vi "Host__MainNewS.vi"() -> ()   [LabVIEW 2018]
uses:
  Type_Def/Type_Def ControlState.ctl
  Type_Def/Type_Def Actuator Controls.ctl
  Type_Def/Master_DataControl.ctl
  Type_Def/TypeDef_cRIODatas.ctl
  Type_Def/Type_Def IMUDatas.ctl
  Type_Def/TypeDef_BMSDatas.ctl
  Type_Def/TypeDef_BMSStatuss.ctl
  Type_Def/TypeDef FixedMotorData.ctl
  <vilib>/Platform/TimedLoop/XDataNode/timing_clust.ctl
  <vilib>/Platform/TimedLoop/XDataNode/nitl_modes.ctl
  <vilib>/Platform/TimedLoop/XDataNode/wakeup.ctl
  <vilib>/Utility/file.llb/Write Delimited Spreadsheet (string).vi
  <vilib>/platform/TimedLoop/XDataNode/XDataNode.xnode
  HealthCheckClass/HealthCheck.lvclass
  <vilib>/Platform/TimedLoop/XDataNode/XDNodeRunTimeDep.lvlib
panel:
  in  "Simulate data":bool
  in  "Simulate Data\nChange values":bool
  out "Fault indicator":bool
  in  "Shutdown":bool
  out "Shorting to\n Chassis":bool
  out "High voltage\nat Contacts":bool
  out "Precharge Indicator":bool
  out "High Side":bool
  out "Vent Indicator":bool
  out "Pump Indicator":bool
  out "Reverse Indicator":bool
  out "Enum":T1
  out "Brake Indicator":bool
  out "Low Side":bool
  out "Forward Indicator":bool
  out "EMCY Brake":bool
  out "24V Power":bool
  out "x Acceleration (g)":dbl(graph)
  out "Speed (mph)":dbl(graph)
  in  "ForceIdle":bool
  in  "stop":bool
  out "HealthCheckTable":string[][](table)
  in  "Tab Control":T2(tab)
  in  "Service Push RPM target":i16=50
  in  "DrvieEnable":bool
  in  "ServiceHOLD":bool
  in  "Service Toggle":bool
  in  "Systems check\nRPM target":i16=50
  in  "Disable Fault \nCheck":bool
  in  "Vent (SC)":bool
  in  "Low Side (SC)":bool
  in  "SystemsCheck enabler":bool caption="High\nSide"
  in  "Brakes (SC)":bool
  in  "Pump (SC)":bool
  in  "Forward (SC)":bool
  in  "Reverse (SC)":bool
  in  "Pre-Charge (SC)":bool
  in  "High Side (SC)":bool
  in  "DriveEnable(SC)":bool
  in  "Release Fault":bool
  in  "Vent":bool
  in  "Ready":bool
  in  "Launch":bool
  out "Braking time (ms)":dbl
  out "Crawling time (ms)":dbl
  out "Crawling Precharge time (ms)":dbl
  out "Pushing time (ms)":dbl
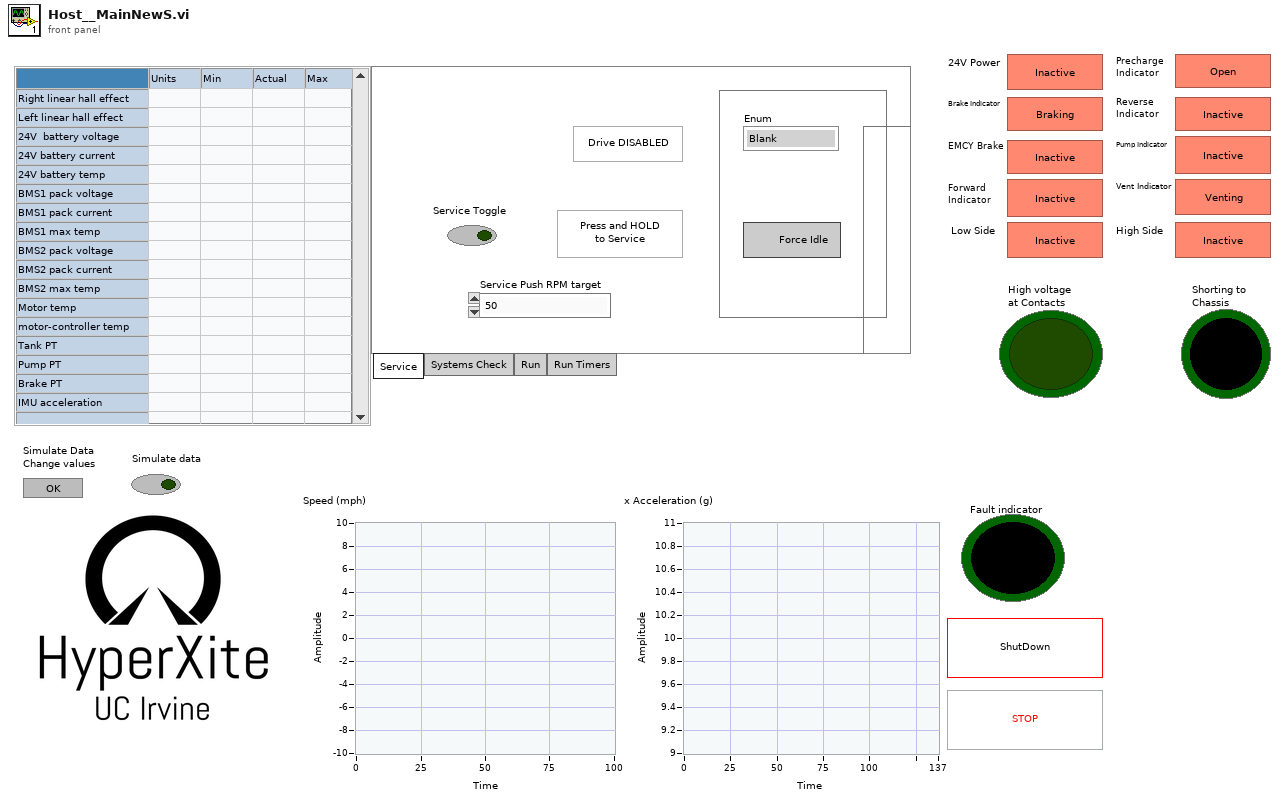
[diagram p1: front panel]
types:
  T1 = typedef "Type_Def ControlState.ctl" = enum16{"Blank", "Systems Check", "Idle", "Ready", "Pushing", "CrawlingPrecharge", "Braking", "Fault", "Boot Up", "Crawling", "Shutdown", "Service Push", "Service Wait", "Vent", "Precharge"}
  T2 = enum32{"Service", "Systems Check", "Run", "Run Timers"}
  T3 = enum8{"Enabled", "Disabled", "Disabled and Grayed Out"}
  T4 = typedef "Type_Def Actuator Controls.ctl" = cluster{"Reverse ":bool, "Precharge Ctrl":bool, "Pump Ctrl":bool, "24 VDC Ctr":bool, "Vent Solenoid":bool, "Brake Solenoid":bool, "EMCY  Brake Solenoid":bool, "Digital Out 7B ":bool, "Forward Ctrl":bool, " Contact H2":bool, "Contact L2":bool, "LED RED":bool, "LED GREEN":bool, " Digital Out 7A":bool, " Contact H1":bool, "Contact L1":bool}
  T5 = typedef "Master_DataControl.ctl" = cluster{"cRIO Data":T6, "IMU Data":T7, "BMS Data":T8, "Motor Data":T10}
  T6 = typedef "TypeDef_cRIODatas.ctl" = cluster{"HallEffect Right (cm)":dbl, "HallEffect Left (cm)":dbl, "Optical Sensor 1 (V)":dbl, "Optical Sensor 2 (V)":dbl, "24V Voltage  (V)":dbl, "24V Current (A)":dbl, "Contactor H1 Continuity":dbl, "Contactor L1 Continuity ":dbl, "Contactor H2 Continuity":dbl, "Contactor L2 Continuity ":dbl, "Brake PT(psig)":dbl, "Pump PT (psig)":dbl, "24V Temp   (C)":dbl, "Tank PT(psig) ":dbl, "ABS Pressure 1 (psig)":dbl, "ABS Pressure 2 (psig) ":dbl, "Displacement (ft)":dbl, "Velocity (ft/s)":dbl, "Time (ms)":dbl, "PV 1 Temp":dbl, "PV2 Temp":dbl}
  T7 = typedef "Type_Def IMUDatas.ctl" = cluster{"y acceleration (g)":dbl, "Pressure (psia)":dbl, "Temperature (F)":dbl}
  T8 = typedef "TypeDef_BMSDatas.ctl" = cluster{"Pack 1 Max Cell\n Voltage (V)":dbl, "Pack 1 Max Cell\n ID ":dbl, "Pack 1 Min Cell \nVoltage (V)":dbl, "Pack 1 Min Cell \nID ":dbl, "Pack 1 State of Charge  (%)":dbl, "Pack 1 Average Voltage1 (V)":dbl, "Pack 1Voltage Delta (V)":dbl, "Pack 1 Current (A)":dbl, "Pack 1 Voltage (V)":dbl, "Pack 1 Max Resistance (Ohm)":dbl, "Pack 1Min Resistance (Ohm)":dbl, "Pack 1Average Resistance (Ohm)":dbl, "Pack 1Delta Resistance (Ohm)":dbl, "Pack 1 Highest Temperature(F)":dbl, "BmsStatus1":T9, "Pack 2 Max Cell\n Voltage (V) ":dbl, "Pack 2 Max Cell\n ID  ":dbl, "Pack 2 Min Cell \nVoltage (V) ":dbl, "Pack 2 Min Cell \nID  ":dbl, "Pack 2 Average Voltage1 (V)":dbl, "Pack 2 Voltage Delta (V) ":dbl, "Pack 2 Current (A)":dbl, "Pack 2 Voltage (V) ":dbl, "Pack 2 State of Charge  (%) ":dbl, "Pack 2 Max Resistance (Ohm) ":dbl, "Pack 2 Min Resistance (Ohm)":dbl, "Pack 2 Average Resistance (Ohm)":dbl, "Pack 2 Delta Resistance (Ohm) ":dbl, "Pack 2 Highest Temperature(F) ":dbl, "BmsStatus 2":T9}
  T9 = typedef "TypeDef_BMSStatuss.ctl" = cluster{"isFault":bool, "isolationMonitoring":bool}
  T10 = typedef "TypeDef FixedMotorData.ctl" = cluster{" Velocity (RPM)":dbl, " MotorTemp(C)":dbl, " ControlTemp(C)":dbl, " DcLinkVolt(V)":dbl, " ErrorCode":dbl, "IsAlive":bool, "motorStatus":cluster{"isReady":bool, "isOn":bool, "isOperEn":bool, "isFault":bool, "isVoltEn":bool, "targetReached":bool, "isWarning":bool}, "motorControllerState":u16}
  T11 = typedef "XDNodeRunTimeDep.lvlib/timing_clust.ctl" = cluster{"Expected End [f-1]":u64, "Actual End [f-1]":u64, "Finished Late? [f-1]":bool, "Expected End [i-1]":u64, "Actual End [i-1]":u64, "Finished Late? [i-1]":bool, "Expected Start [i]":u64, "Actual Start [i]":u64, "Expected Start [f]":u64, "Actual Start [f]":u64, "Source Name":string, "Structure Name":string, "Period":i64, "Deadline":i64, "Offset":i64, "Start":i64, "Priority":i32, "Timeout":i32, "Mode":T12, "Wakeup Reason":T13, "Error":errorcluster, "Source Type":string, "Secondary Source Type":string, "Global End Time":u64, "Global Start Time":u64, "Frame Duration":u64, "Iteration Duration":u64, "Assigned CPU":i32, "I/O Scan Engine Mode":u32}
  T12 = typedef "XDNodeRunTimeDep.lvlib/nitl_modes.ctl" = enum32{"No Change", "Process missed periods, maintain original phase", "Discard missed periods, maintain original phase", "Process missed periods, ignore original phase", "Discard missed periods, ignore original phase"}
  T13 = typedef "XDNodeRunTimeDep.lvlib/wakeup.ctl" = enum32{"Normal", "Aborted", "Asynchronous wakeup", "Timing source error", "Timed loop error", "Timeout"}
  T14 = typedef "HealthCheck.lvclass/HCState_TypeDef.ctl" = enum16{"Initialization", "Running", "Modify Table"}
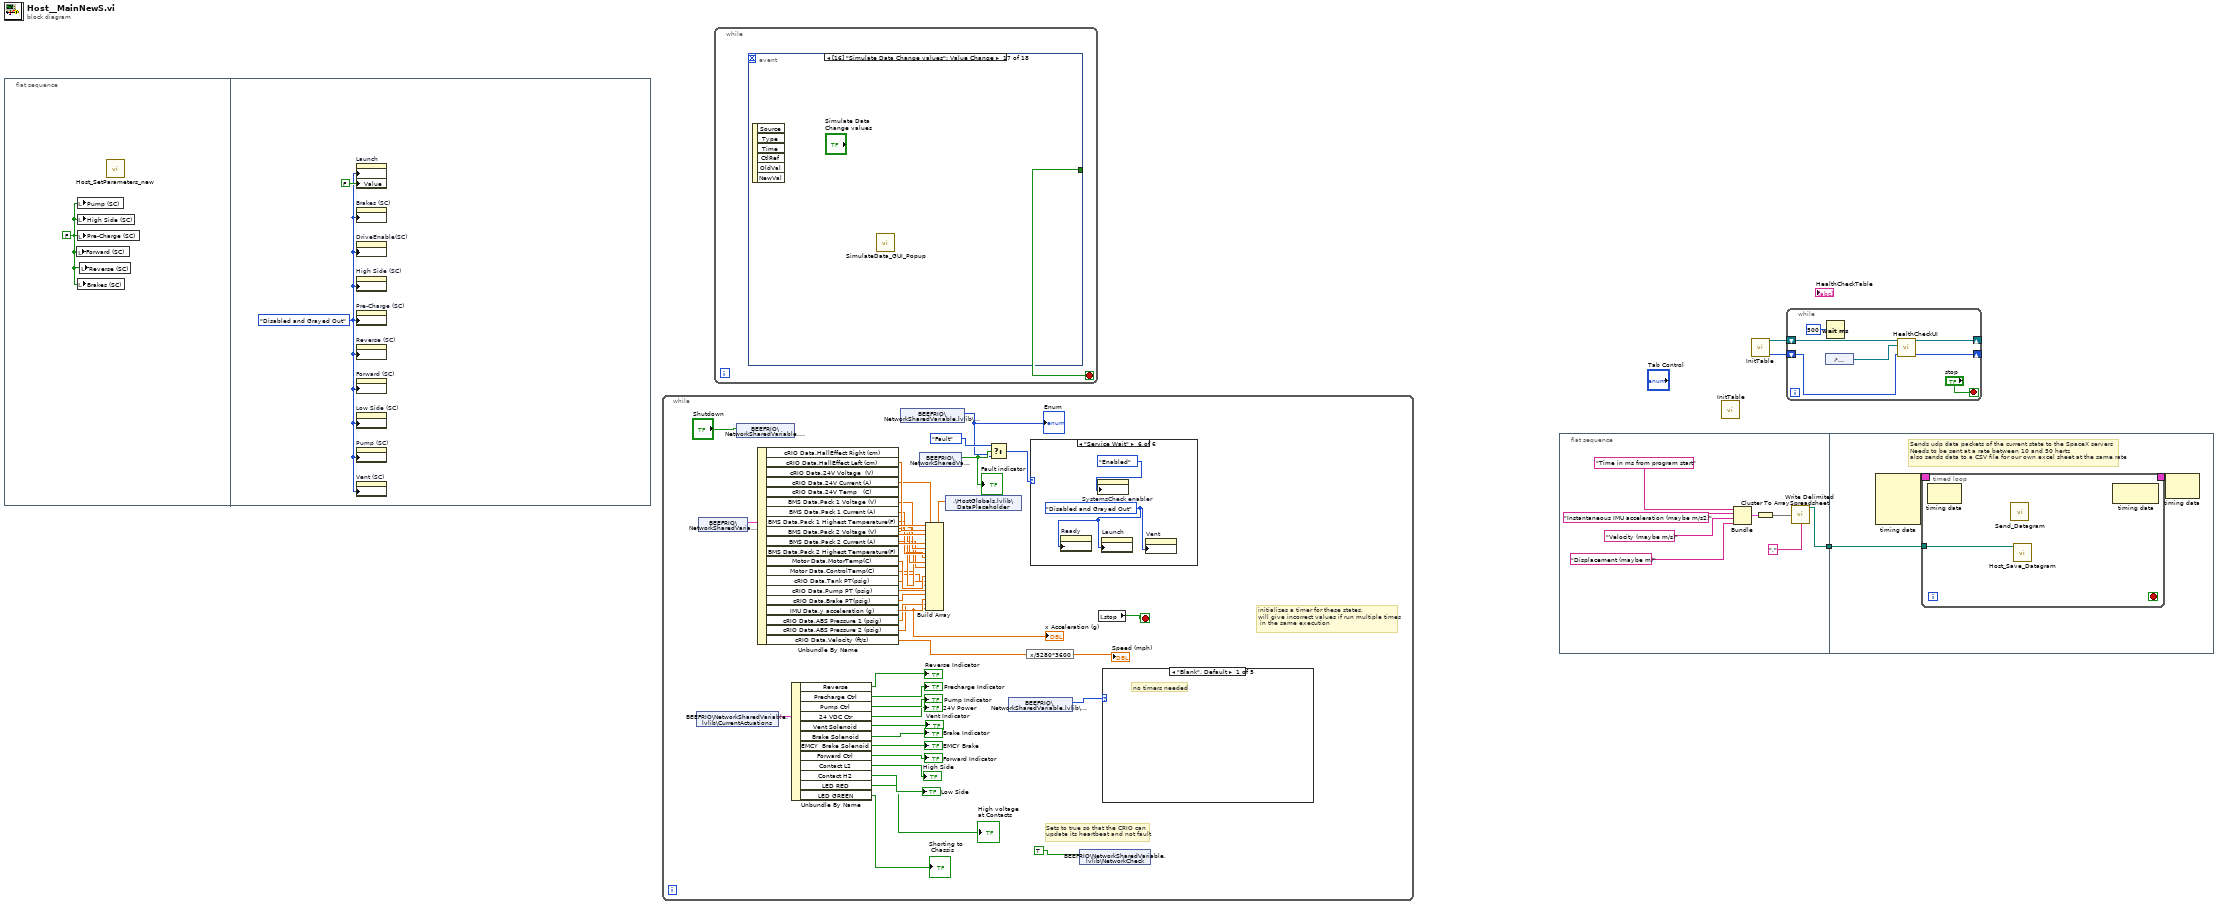
[diagram p0: block diagram]
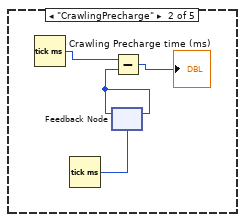
[diagram p2: hidden frame]
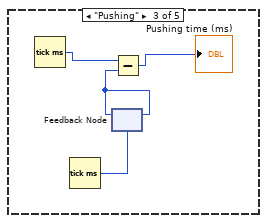
[diagram p3: hidden frame]
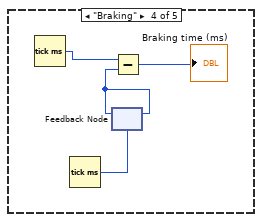
[diagram p4: hidden frame]
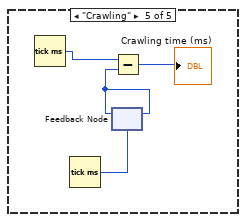
[diagram p5: hidden frame]
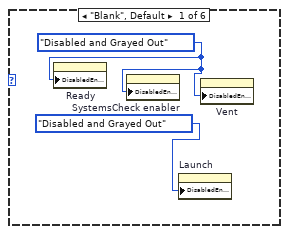
[diagram p6: hidden frame]
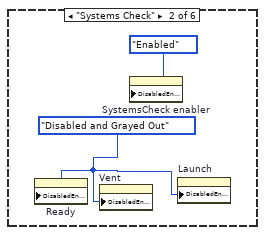
[diagram p7: hidden frame]
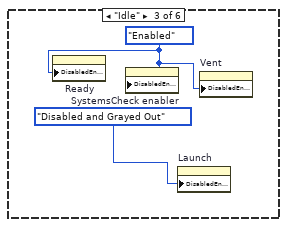
[diagram p8: hidden frame]
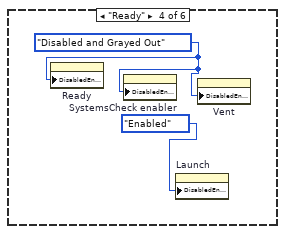
[diagram p9: hidden frame]
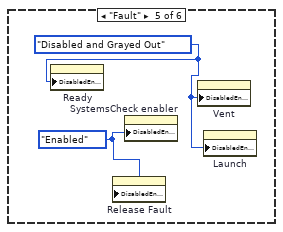
[diagram p10: hidden frame]
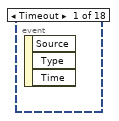
[diagram p11: hidden frame]
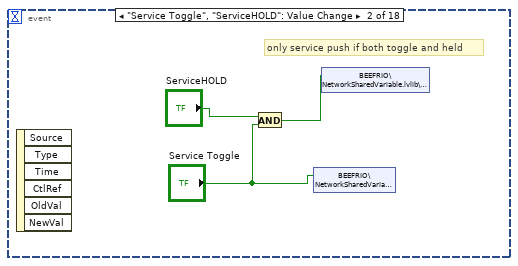
[diagram p12: hidden frame]
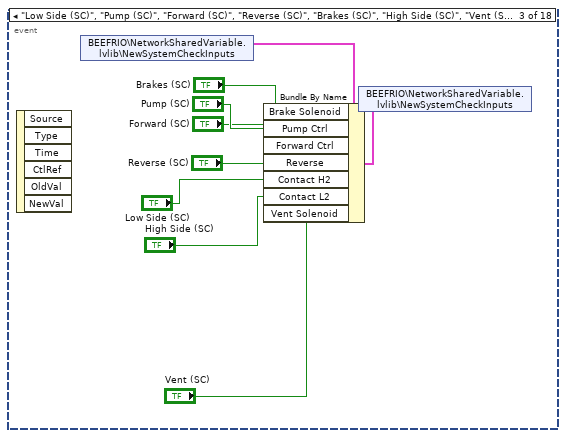
[diagram p13: hidden frame]
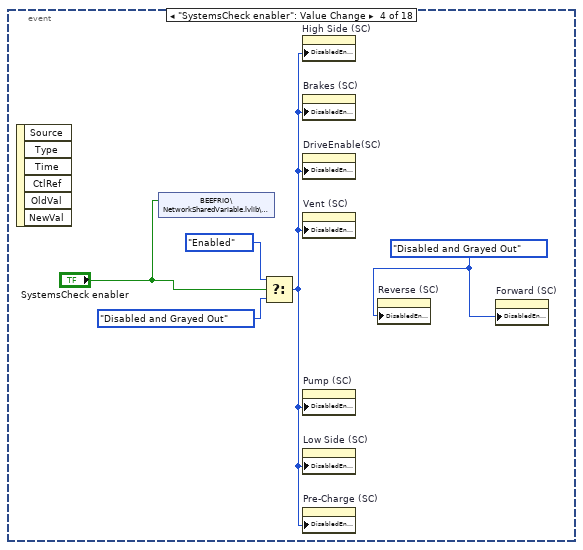
[diagram p14: hidden frame]
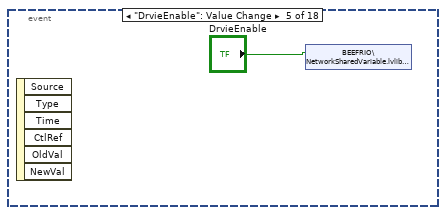
[diagram p15: hidden frame]
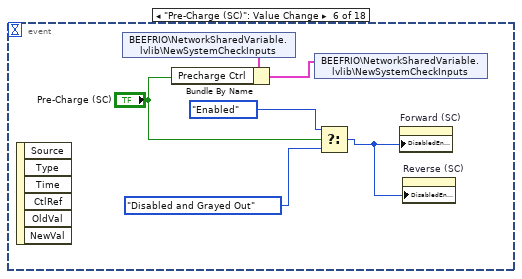
[diagram p16: hidden frame]
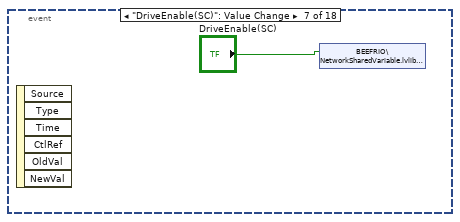
[diagram p17: hidden frame]
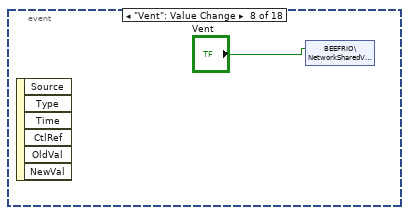
[diagram p18: hidden frame]
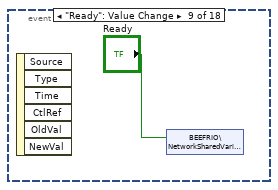
[diagram p19: hidden frame]
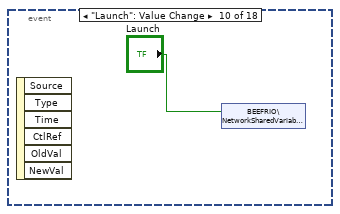
[diagram p20: hidden frame]
diagram:
  n1 = flat-sequence {
    frame #0 {
      w4 = FALSE
      n2 = local write "Forward (SC)"(w4) -> ()
      n3 = local write "Pump (SC)"(w4) -> ()
      n4 = local write "High Side (SC)"(w4) -> ()
      n5 = local write "Pre-Charge (SC)"(w4) -> ()
      n6 = local write "Brakes (SC)"(w4) -> ()
      n7 = local write "Reverse (SC)"(w4) -> ()
      n8 = call "Host_SetParameters_new.vi"() -> ()  [unwired: 12 in]
    }
    frame #1 {
      w5 = T3."Disabled and Grayed Out" ("Disabled")
      n9 = property on="Launch" class="Bool"("DisabledEnum"=w5, "Value"=FALSE) -> ()  [unwired: 2 in, 2 out]
      n10 = property on="Brakes (SC)" class="Bool (strict)"("DisabledEnum"=w5) -> ()  [unwired: 2 in, 2 out]
      n11 = property on="DriveEnable(SC)" class="Bool (strict)"("DisabledEnum"=w5) -> ()  [unwired: 2 in, 2 out]
      n12 = property on="High Side (SC)" class="Bool (strict)"("DisabledEnum"=w5) -> ()  [unwired: 2 in, 2 out]
      n13 = property on="Pre-Charge (SC)" class="Bool (strict)"("DisabledEnum"=w5) -> ()  [unwired: 2 in, 2 out]
      n14 = property on="Reverse (SC)" class="Bool (strict)"("DisabledEnum"=w5) -> ()  [unwired: 2 in, 2 out]
      n15 = property on="Forward (SC)" class="Bool (strict)"("DisabledEnum"=w5) -> ()  [unwired: 2 in, 2 out]
      n16 = property on="Low Side (SC)" class="Bool (strict)"("DisabledEnum"=w5) -> ()  [unwired: 2 in, 2 out]
      n17 = property on="Pump (SC)" class="Bool (strict)"("DisabledEnum"=w5) -> ()  [unwired: 2 in, 2 out]
      n18 = property on="Vent (SC)" class="Bool (strict)"("DisabledEnum"=w5) -> ()  [unwired: 2 in, 2 out]
    }
  }
  n19 = while {
    stop <- w49 stop-if-true
    # "initializes a timer for these states,\nwill give incorrect values if run multiple times\n in the same execution"
    # "Sets to true so that the CRIO can \nupdate its heartbeat and not fault"
    n20 = shared-variable "BEEFRIO\\NetworkSharedVariable.lvlib\\CurrentActuations"() -> (w46:T4)  [unwired: 1 in, 1 out]
    n21 = shared-variable "BEEFRIO\\NetworkSharedVariable.lvlib\\AllData"() -> (w50:T5)  [unwired: 1 in, 1 out]
    n22 = shared-variable "BEEFRIO\\NetworkSharedVariable.lvlib\\Shutdown"("Shutdown") -> ()  [unwired: 1 in, 1 out]
    n23 = Unbundle By Name(w50) -> ("cRIO Data.HallEffect Right (cm)"=w34:dbl, "cRIO Data.HallEffect Left (cm)"=w33:dbl, "cRIO Data.24V Voltage  (V)"=w32:dbl, "cRIO Data.24V Current (A)"=w31:dbl, "cRIO Data.24V Temp   (C)"=w30:dbl, "BMS Data.Pack 1 Voltage (V)"=w28:dbl, "BMS Data.Pack 1 Current (A)"=w27:dbl, "BMS Data.Pack 1 Highest Temperature(F)"=w26:dbl, "BMS Data.Pack 2 Voltage (V)"=w25:dbl, "BMS Data.Pack 2 Current (A)"=w24:dbl, "BMS Data.Pack 2 Highest Temperature(F)"=w23:dbl, "Motor Data.MotorTemp(C)"=w22:dbl, "Motor Data.ControlTemp(C)"=w21:dbl, "cRIO Data.Tank PT(psig)"=w20:dbl, "cRIO Data.Pump PT (psig)"=w19:dbl, "cRIO Data.Brake PT(psig)"=w18:dbl, "IMU Data.y acceleration (g)"=w17:dbl, "cRIO Data.ABS Pressure 1 (psig)"=w16:dbl, "cRIO Data.ABS Pressure 2 (psig)"=w15:dbl, "cRIO Data.Velocity (ft/s)"=w48:dbl)
    "x Acceleration (g)" <- w17
    n24 = Unbundle By Name(w46) -> ("Reverse"=→"Reverse Indicator":bool, "Precharge Ctrl"=→"Precharge Indicator":bool, "Pump Ctrl"=→"Pump Indicator":bool, "24 VDC Ctr"=→"24V Power":bool, "Vent Solenoid"=→"Vent Indicator":bool, "Brake Solenoid"=→"Brake Indicator":bool, "EMCY  Brake Solenoid"=→"EMCY Brake":bool, "Forward Ctrl"=→"Forward Indicator":bool, "Contact L2"=→"High Side":bool, "Contact H2"=→"Low Side":bool, "LED RED"=→"High voltage\nat Contacts":bool, "LED GREEN"=→"Shorting to\n Chassis":bool)
    n25 = shared-variable "BEEFRIO\\NetworkSharedVariable.lvlib\\CurrentState"() -> (w10:T1)  [unwired: 1 in, 1 out]
    "Enum" <- w10
    n26 = shared-variable "BEEFRIO\\NetworkSharedVariable.lvlib\\Fault"() -> (w13:bool)  [unwired: 1 in, 1 out]
    "Fault indicator" <- w13
    n27 = Build Array(w34, w33, w32, w31, w30, w28, w27, w26, w25, w24, w23, w22, w21, w20, w19, w18, w17, w16, w15) -> (w29:dbl[])
    n28 = shared-variable ".\\HostGlobals.lvlib\\DataPlaceholder"(w29) -> ()  [unwired: 1 in, 1 out]
    n29 = Select(t=Type_Def_ControlState."Fault" ("CurrentState"), s=w13, f=w10) -> (s? t:f=w11:T1)
    n30 = shared-variable "BEEFRIO\\NetworkSharedVariable.lvlib\\CurrentState"() -> (w9:T1)  [unwired: 1 in, 1 out]
    n31 = expression code="x/5280*3600"(w48) -> (→"Speed (mph)":dbl)
    n32 = case shown="\"Service Wait\"" w11 {
      frame "Blank", Default {
        w68 = T3."Disabled and Grayed Out" ("Disabled")
        n33 = property on="Ready" class="Bool"("DisabledEnum"=w68) -> ()  [unwired: 2 in, 2 out]
        n34 = property on="SystemsCheck enabler" class="Bool (strict)"("DisabledEnum"=w68) -> ()  [unwired: 2 in, 2 out]
        n35 = property on="Launch" class="Bool"("DisabledEnum"=T3."Disabled and Grayed Out" ("Disabled")) -> ()  [unwired: 2 in, 2 out]
        n36 = property on="Vent" class="Bool"("DisabledEnum"=w68) -> ()  [unwired: 2 in, 2 out]
      }
      frame "Systems Check" {
        w69 = T3."Disabled and Grayed Out" ("Disabled")
        n37 = property on="Ready" class="Bool"("DisabledEnum"=w69) -> ()  [unwired: 2 in, 2 out]
        n38 = property on="Vent" class="Bool"("DisabledEnum"=w69) -> ()  [unwired: 2 in, 2 out]
        n39 = property on="SystemsCheck enabler" class="Bool (strict)"("DisabledEnum"=T3."Enabled" ("Disabled")) -> ()  [unwired: 2 in, 2 out]
        n40 = property on="Launch" class="Bool"("DisabledEnum"=w69) -> ()  [unwired: 2 in, 2 out]
      }
      frame "Idle" {
        w71 = T3."Enabled" ("Disabled")
        n41 = property on="Ready" class="Bool"("DisabledEnum"=w71) -> ()  [unwired: 2 in, 2 out]
        n42 = property on="SystemsCheck enabler" class="Bool (strict)"("DisabledEnum"=w71) -> ()  [unwired: 2 in, 2 out]
        n43 = property on="Launch" class="Bool"("DisabledEnum"=T3."Disabled and Grayed Out" ("Disabled")) -> ()  [unwired: 2 in, 2 out]
        n44 = property on="Vent" class="Bool"("DisabledEnum"=w71) -> ()  [unwired: 2 in, 2 out]
      }
      frame "Ready" {
        w74 = T3."Disabled and Grayed Out" ("Disabled")
        n45 = property on="Ready" class="Bool"("DisabledEnum"=w74) -> ()  [unwired: 2 in, 2 out]
        n46 = property on="SystemsCheck enabler" class="Bool (strict)"("DisabledEnum"=w74) -> ()  [unwired: 2 in, 2 out]
        n47 = property on="Launch" class="Bool"("DisabledEnum"=T3."Enabled" ("Disabled")) -> ()  [unwired: 2 in, 2 out]
        n48 = property on="Vent" class="Bool"("DisabledEnum"=w74) -> ()  [unwired: 2 in, 2 out]
      }
      frame "Fault" {
        w75 = T3."Enabled" ("Disabled")
        w76 = T3."Disabled and Grayed Out" ("Disabled")
        n49 = property on="Ready" class="Bool"("DisabledEnum"=w76) -> ()  [unwired: 2 in, 2 out]
        n50 = property on="Release Fault" class="Bool"("DisabledEnum"=w75) -> ()  [unwired: 2 in, 2 out]
        n51 = property on="SystemsCheck enabler" class="Bool (strict)"("DisabledEnum"=w75) -> ()  [unwired: 2 in, 2 out]
        n52 = property on="Vent" class="Bool"("DisabledEnum"=w76) -> ()  [unwired: 2 in, 2 out]
        n53 = property on="Launch" class="Bool"("DisabledEnum"=w76) -> ()  [unwired: 2 in, 2 out]
      }
      frame "Service Wait" {
        w77 = T3."Disabled and Grayed Out" ("Disabled")
        n54 = property on="Ready" class="Bool"("DisabledEnum"=w77) -> ()  [unwired: 2 in, 2 out]
        n55 = property on="SystemsCheck enabler" class="Bool (strict)"("DisabledEnum"=T3."Enabled" ("Disabled")) -> ()  [unwired: 2 in, 2 out]
        n56 = property on="Launch" class="Bool"("DisabledEnum"=w77) -> ()  [unwired: 2 in, 2 out]
        n57 = property on="Vent" class="Bool"("DisabledEnum"=w77) -> ()  [unwired: 2 in, 2 out]
      }
    }
    n58 = shared-variable "BEEFRIO\\NetworkSharedVariable.lvlib\\NetworkCheck"(TRUE) -> ()  [unwired: 1 in, 1 out]
    n59 = local read "stop"() -> (w49:bool)
    n60 = case shown="\"Blank\", Default" w9 {
      frame "Blank", Default {
        # "no timers needed"
      }
      frame "CrawlingPrecharge" {
        n61 = Tick Count (ms)() -> (millisecond timer value=w54:u32)
        n62 = Tick Count (ms)() -> (millisecond timer value=w53:u32)
        n63 = feedback #1(w53) -> (w52:u32)
        n64 = feedback-in #1(w52) -> ()
        n65 = Subtract(x=w54, y=w52) -> (x-y=→"Crawling Precharge time (ms)":u32)
      }
      frame "Pushing" {
        n66 = Tick Count (ms)() -> (millisecond timer value=w58:u32)
        n67 = Tick Count (ms)() -> (millisecond timer value=w57:u32)
        n68 = feedback #2(w57) -> (w55:u32)
        n69 = feedback-in #2(w55) -> ()
        n70 = Subtract(x=w58, y=w55) -> (x-y=→"Pushing time (ms)":u32)
      }
      frame "Braking" {
        n71 = Tick Count (ms)() -> (millisecond timer value=w62:u32)
        n72 = Tick Count (ms)() -> (millisecond timer value=w61:u32)
        n73 = feedback #3(w61) -> (w60:u32)
        n74 = feedback-in #3(w60) -> ()
        n75 = Subtract(x=w62, y=w60) -> (x-y=→"Braking time (ms)":u32)
      }
      frame "Crawling" {
        n76 = Tick Count (ms)() -> (millisecond timer value=w66:u32)
        n77 = Tick Count (ms)() -> (millisecond timer value=w65:u32)
        n78 = feedback #4(w65) -> (w64:u32)
        n79 = feedback-in #4(w64) -> ()
        n80 = Subtract(x=w66, y=w64) -> (x-y=→"Crawling time (ms)":u32)
      }
    }
  }
  n81 = while {
    stop <- w79 stop-if-true
    n82 = event shown="[16] \"Simulate Data Change values\": Value Change" {
      selector: _ -> [_ _ _ _ _ _ _ _ _ _ _ _ _ _ _ _ _ _]
      dyn-events: _ -> [_ _ _ _ _ _ _ _ _ _ _ _ _ _ _ _ _ _]
      timeout: _ -> [_ _ _ _ _ _ _ _ _ _ _ _ _ _ _ _ _ _]
      tunnel: [_ _ _ _ _ _ _ _ _ _ _ _ w110 _ _ _ _ _] -> w79
      event Timeout {
        n83 = event-data() -> ()  [unwired: 1 in, 3 out]
      }
      event "Service Toggle", "ServiceHOLD": Value Change {
        # "only service push if both toggle and held"
        n84 = event-data() -> ()  [unwired: 1 in, 6 out]
        n85 = And(x="ServiceHOLD", y="Service Toggle") -> (x .and. y?=w82:bool)
        n86 = shared-variable "BEEFRIO\\NetworkSharedVariable.lvlib\\Service"("Service Toggle") -> ()  [unwired: 1 in, 1 out]
        n87 = shared-variable "BEEFRIO\\NetworkSharedVariable.lvlib\\ServicePush"(w82) -> ()  [unwired: 1 in, 1 out]
      }
      event "Low Side (SC)", "Pump (SC)", "Forward (SC)", "Reverse (SC)", "Brakes (SC)", "High Side (SC)", "Vent (SC)": Value Change {
        n88 = event-data() -> ()  [unwired: 1 in, 6 out]
        n89 = shared-variable "BEEFRIO\\NetworkSharedVariable.lvlib\\NewSystemCheckInputs"() -> (w86:T4)  [unwired: 1 in, 1 out]
        n90 = Bundle By Name(cluster=w86, "Brake Solenoid"="Brakes (SC)", "Pump Ctrl"="Pump (SC)", "Forward Ctrl"="Forward (SC)", "Reverse"="Reverse (SC)", "Contact H2"="Low Side (SC)", "Contact L2"="High Side (SC)", "Vent Solenoid"="Vent (SC)") -> (w87:T4)
        n91 = shared-variable "BEEFRIO\\NetworkSharedVariable.lvlib\\NewSystemCheckInputs"(w87) -> ()  [unwired: 1 in, 1 out]
      }
      event "SystemsCheck enabler": Value Change {
        w94 = T3."Disabled and Grayed Out" ("Disabled")
        n92 = event-data() -> ()  [unwired: 1 in, 6 out]
        n93 = shared-variable "BEEFRIO\\NetworkSharedVariable.lvlib\\SystemCheck"("SystemsCheck enabler") -> ()  [unwired: 1 in, 1 out]
        n94 = Select(t=T3."Enabled" ("Disabled"), s="SystemsCheck enabler", f=T3."Disabled and Grayed Out" ("Disabled")) -> (s? t:f=w93:T3)
        n95 = property on="High Side (SC)" class="Bool (strict)"("DisabledEnum"=w93) -> ()  [unwired: 2 in, 2 out]
        n96 = property on="Brakes (SC)" class="Bool (strict)"("DisabledEnum"=w93) -> ()  [unwired: 2 in, 2 out]
        n97 = property on="DriveEnable(SC)" class="Bool (strict)"("DisabledEnum"=w93) -> ()  [unwired: 2 in, 2 out]
        n98 = property on="Vent (SC)" class="Bool (strict)"("DisabledEnum"=w93) -> ()  [unwired: 2 in, 2 out]
        n99 = property on="Pump (SC)" class="Bool (strict)"("DisabledEnum"=w93) -> ()  [unwired: 2 in, 2 out]
        n100 = property on="Low Side (SC)" class="Bool (strict)"("DisabledEnum"=w93) -> ()  [unwired: 2 in, 2 out]
        n101 = property on="Pre-Charge (SC)" class="Bool (strict)"("DisabledEnum"=w93) -> ()  [unwired: 2 in, 2 out]
        n102 = property on="Reverse (SC)" class="Bool (strict)"("DisabledEnum"=w94) -> ()  [unwired: 2 in, 2 out]
        n103 = property on="Forward (SC)" class="Bool (strict)"("DisabledEnum"=w94) -> ()  [unwired: 2 in, 2 out]
      }
      event "DrvieEnable": Value Change {
        n104 = event-data() -> ()  [unwired: 1 in, 6 out]
        n105 = shared-variable "BEEFRIO\\NetworkSharedVariable.lvlib\\driveEnable"("DrvieEnable") -> ()  [unwired: 1 in, 1 out]
      }
      event "Pre-Charge (SC)": Value Change {
        n106 = event-data() -> ()  [unwired: 1 in, 6 out]
        n107 = shared-variable "BEEFRIO\\NetworkSharedVariable.lvlib\\NewSystemCheckInputs"() -> (w103:T4)  [unwired: 1 in, 1 out]
        n108 = Bundle By Name(cluster=w103, "Precharge Ctrl"="Pre-Charge (SC)") -> (w102:T4)
        n109 = shared-variable "BEEFRIO\\NetworkSharedVariable.lvlib\\NewSystemCheckInputs"(w102) -> ()  [unwired: 1 in, 1 out]
        n110 = Select(t=T3."Enabled" ("Disabled"), s="Pre-Charge (SC)", f=T3."Disabled and Grayed Out" ("Disabled")) -> (s? t:f=w98:T3)
        n111 = property on="Forward (SC)" class="Bool (strict)"("DisabledEnum"=w98) -> ()  [unwired: 2 in, 2 out]
        n112 = property on="Reverse (SC)" class="Bool (strict)"("DisabledEnum"=w98) -> ()  [unwired: 2 in, 2 out]
      }
      event "DriveEnable(SC)": Value Change {
        n113 = event-data() -> ()  [unwired: 1 in, 6 out]
        n114 = shared-variable "BEEFRIO\\NetworkSharedVariable.lvlib\\driveEnable"("DriveEnable(SC)") -> ()  [unwired: 1 in, 1 out]
      }
      event "Vent": Value Change {
        n115 = event-data() -> ()  [unwired: 1 in, 6 out]
        n116 = shared-variable "BEEFRIO\\NetworkSharedVariable.lvlib\\Vent"("Vent") -> ()  [unwired: 1 in, 1 out]
      }
      event "Ready": Value Change {
        n117 = event-data() -> ()  [unwired: 1 in, 6 out]
        n118 = shared-variable "BEEFRIO\\NetworkSharedVariable.lvlib\\Ready"("Ready") -> ()  [unwired: 1 in, 1 out]
      }
      event "Launch": Value Change {
        n119 = event-data() -> ()  [unwired: 1 in, 6 out]
        n120 = shared-variable "BEEFRIO\\NetworkSharedVariable.lvlib\\Launch"("Launch") -> ()  [unwired: 1 in, 1 out]
      }
      event "Release Fault": Value Change {
        n121 = event-data() -> ()  [unwired: 1 in, 6 out]
        n122 = shared-variable "BEEFRIO\\NetworkSharedVariable.lvlib\\Fault"(FALSE) -> ()  [unwired: 1 in, 1 out]
      }
      event "ForceIdle": Value Change {
        n123 = event-data() -> ()  [unwired: 1 in, 6 out]
        n124 = shared-variable "BEEFRIO\\NetworkSharedVariable.lvlib\\ForceIdle"("ForceIdle") -> ()  [unwired: 1 in, 1 out]
      }
      event "stop": Value Change {
        n125 = event-data() -> ()  [unwired: 1 in, 6 out]
        n126 = local read "stop"() -> (w110:bool)
      }
      event "Disable Fault \nCheck": Value Change {
        n127 = event-data() -> ()  [unwired: 1 in, 6 out]
        n128 = shared-variable "BEEFRIO\\NetworkSharedVariable.lvlib\\DisableFaultCheck"("Disable Fault \nCheck") -> ()  [unwired: 1 in, 1 out]
      }
      event "Service Push RPM target": Value Change {
        n129 = event-data() -> ()  [unwired: 1 in, 6 out]
        n130 = shared-variable "BEEFRIO\\NetworkSharedVariable.lvlib\\ServiceRPMTarget"("Service Push RPM target") -> ()  [unwired: 1 in, 1 out]
      }
      event "Systems check\nRPM target": Value Change {
        n131 = event-data() -> ()  [unwired: 1 in, 6 out]
        n132 = shared-variable "BEEFRIO\\NetworkSharedVariable.lvlib\\SystemCheckRPMTarget"("Systems check\nRPM target") -> ()  [unwired: 1 in, 1 out]
      }
      event "Simulate Data\nChange values": Value Change {
        n133 = event-data() -> ()  [unwired: 1 in, 6 out]
        n134 = call "SimulateData_GUI_Popup.vi"() -> ()  [unwired: 12 in]
      }
      event "Simulate data": Value Change {
        n135 = event-data() -> ()  [unwired: 1 in, 6 out]
        n136 = shared-variable "BEEFRIO\\NetworkSharedVariable.lvlib\\SimulateData"("Simulate data") -> ()  [unwired: 1 in, 1 out]
      }
    }
  }
  n137 = flat-sequence {
    tunnel: [w115] -> w1
    tunnel: w1 -> [w123]
    frame #0 {
      n138 = Bundle("Time in ms from program start", "Instantaneous IMU acceleration (maybe m/s2)", "Velocity (maybe m/s)", "Displacement (maybe m)") -> (w122:cluster{string, string, string, string})  [unwired: 1 in]
      n139 = Cluster To Array(cluster=w122) -> (array=w121:string[])
      n140 = call-poly <vilib>:"Write Delimited Spreadsheet.vi"("1D data"=w121, "delimiter (\\t)"=",") -> ("new file path (Not A Path if cancelled)"=w115:path)  [unwired: 12 in, 1 out]
    }
    frame #1 {
      # "Sends udp data packets of the current state to the SpaceX servers\nNeeds to be sent at a rate between 10 and 50 hertz\nalso sends data to a CSV file for our own excel sheet at the same rate"
      n141 = node-c288() -> (w125:T11)  [unwired: 4 in]
      n142 = timed-loop {
        timing: w125 -> [_]
        timing-out: [_] -> w124
        tunnel: w123 -> [w126]
        stop <- _ stop-if-true
        n143 = node-c288() -> ()  [unwired: 1 in, 1 out]
        n144 = call "Send_Datagram.vi"() -> ()  [unwired: 12 in]
        n145 = call "Host_Save_Datagram.vi"("Path"=w126) -> ()  [unwired: 11 in]
        n146 = node-c288() -> ()  [unwired: 1 in, 1 out]
      }
      n147 = node-c288(w124) -> ()  [unwired: 1 out]
    }
  }
  n148 = call "InitTable.vi"() -> ()  [unwired: 10 in, 2 out]
  n149 = call "InitTable.vi"() -> ("Enum out"=w2:T14, "HealthCheck out"=w3:refnum<class "HealthCheck.lvclass">)  [unwired: 10 in]
  n150 = while {
    shift-right: [w134] -> _
    shift-left: w3 -> [w133]
    shift-right: [w132] -> _
    shift-left: w2 -> [w131]
    stop <- "stop" stop-if-true
    n151 = control-ref of="HealthCheckTable"() -> (w135:refnum<vi>)
    n152 = Wait (ms)(milliseconds to wait=u32 500) -> ()  [unwired: 1 out]
    n153 = call "HealthCheckUI.vi"("Enum in"=w131, "Table in"=w135, "HealthCheck.lvclass"=w133) -> ("Enum out"=w132:T14, "HealthCheck out"=w134:refnum<class "HealthCheck.lvclass">)  [unwired: 7 in]
  }
